vi "AttackHim.vi"(8 "error in (no error)":errorcluster, 9 "Cube":i32, 10 "Rival":refnum<class "Peasant.lvclass">, 11 "Peasant in":refnum<class "Peasant.lvclass">) -> (0 "error out":errorcluster, 1 "CurrentAttack":i32, 2 "Rival out":refnum<class "Peasant.lvclass">, 3 "Peasant out":refnum<class "Peasant.lvclass">)   [LabVIEW 2021, in "Peasant.lvclass"]
uses:
  Peasant.lvclass
  Peasant.lvclass/Peasant.ctl
  Accessory/Accessory.lvclass
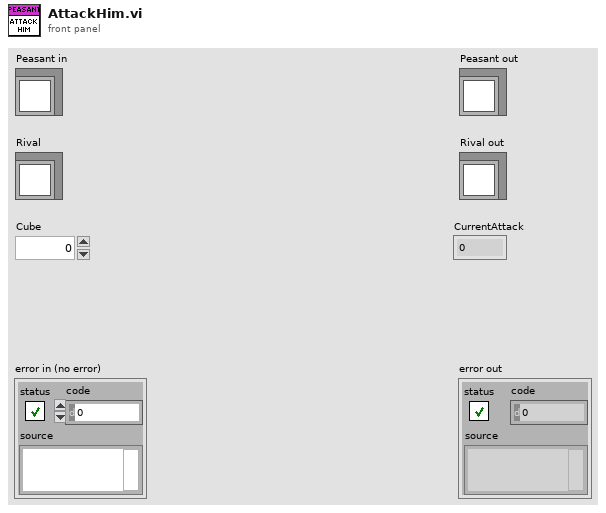
[diagram p1: front panel]
types:
  T1 = typedef "Peasant.lvclass/PeasantAttributes.ctl" = cluster{"Health":i32, "Stamina":i32, "Attack":i32, "Defense":i32, "Sing":i32}
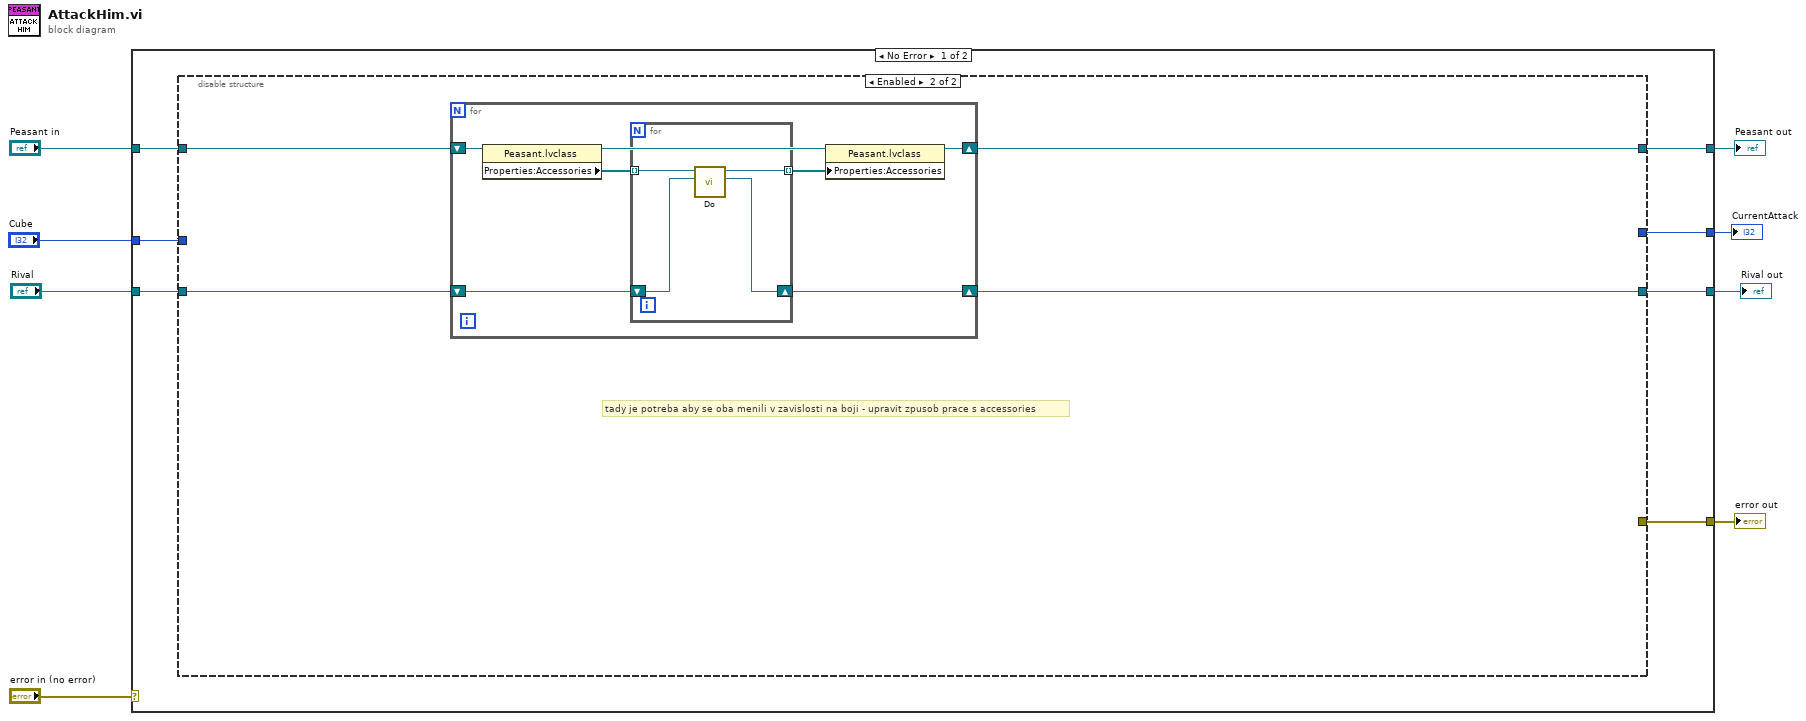
[diagram p0: block diagram]
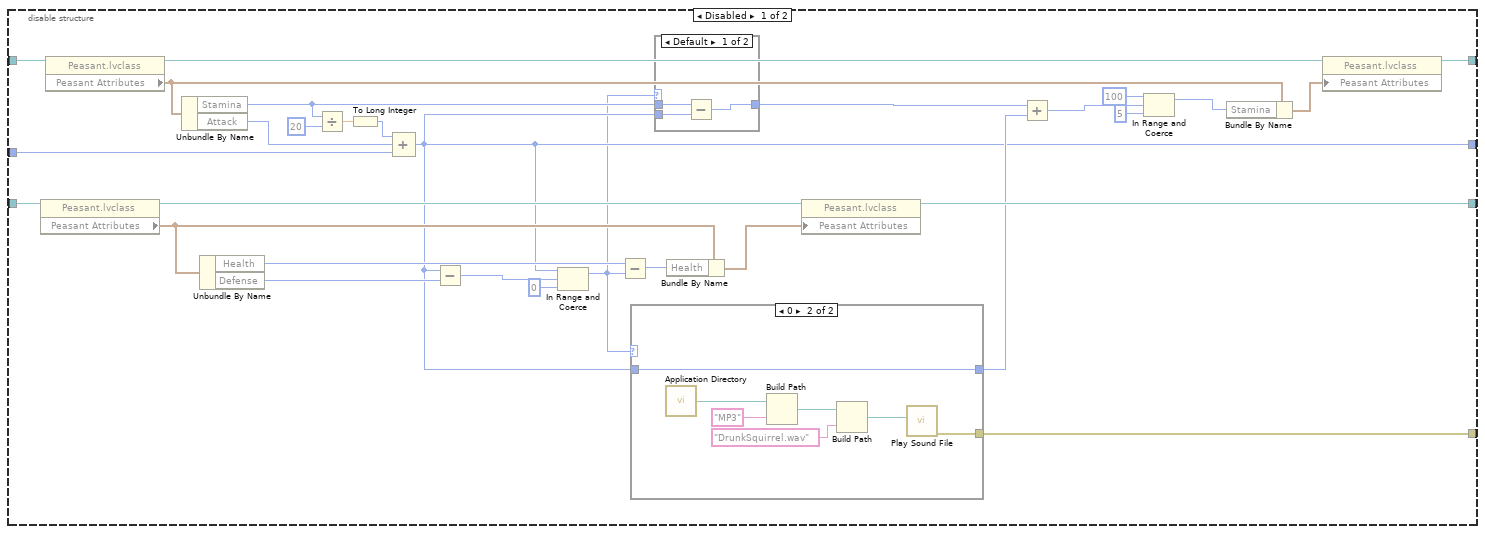
[diagram p2: hidden frame]
diagram:
  n1 = case shown="No Error" "error in (no error)" {
    selector: "error in (no error)" -> [_ w74]
    tunnel: [w11 w74] -> w7
    tunnel: [w12 w73] -> w5
    tunnel: "Peasant in" -> [w15 w73]
    tunnel: "Rival" -> [w14 w72]
    tunnel: "Cube" -> [w10 _]
    tunnel: [w13 w72] -> w2
    tunnel: [w9 _] -> w1
    frame No Error {
      n2 = disable-structure shown="Enabled" {
        disable-tunnel: w15 -> [w45 w60]
        disable-tunnel: w14 -> [w44 w59]
        disable-tunnel: [w38 w58] -> w13
        disable-tunnel: [w31 w57] -> w12
        disable-tunnel: [w30 _] -> w11
        disable-tunnel: w10 -> [w23 _]
        disable-tunnel: [w18 _] -> w9
        frame Disabled {
          n3 = property class="Peasant.lvclass"(reference=w44) -> (reference out=w40:refnum<class "Peasant.lvclass">, "Peasant Attributes"=w42:T1)  [unwired: 1 in, 1 out]
          n4 = property class="Peasant.lvclass"(reference=w45) -> (reference out=w34:refnum<class "Peasant.lvclass">, "Peasant Attributes"=w33:T1)  [unwired: 1 in, 1 out]
          n5 = Unbundle By Name(w33) -> ("Stamina"=w22:i32, "Attack"=w24:i32)
          n6 = Unbundle By Name(w42) -> ("Health"=w43:i32, "Defense"=w37:i32)
          n7 = Divide(x=w22, y=20) -> (x/y=w20:dbl)
          n8 = To Long Integer(number=w20) -> (32bit integer=w19:i32)
          n9 = Compound Arithmetic op=ADD(w19, w24, w23) -> (w18:i32)
          n10 = Subtract(x=w18, y=w37) -> (x-y=w35:i32)
          n11 = In Range and Coerce(upper limit=w18, x=w35, lower limit=0) -> (coerced(x)=w16:i32)  [unwired: 1 out]
          n12 = Subtract(x=w43, y=w16) -> (x-y=w41:i32)
          n13 = case shown="0" w16 {
            tunnel: [_ w51] -> w30
            tunnel: w18 -> [_ w50]
            tunnel: [_ w50] -> w28
            frame Default {
            }
            frame 0 {
              n14 = call <vilib>:"Application Directory.vi"() -> ("Application Directory"=w56:path)
              n15 = Build Path(base path=w56, name or relative path="MP3") -> (appended path=w54:path)
              n16 = Build Path(base path=w54, name or relative path="DrunkSquirrel.wav") -> (appended path=w52:path)
              n17 = call <vilib>:"Play Sound File.vi"("path"=w52) -> ("error out"=w51:errorcluster)  [unwired: 9 in, 1 out]
            }
          }
          n18 = case shown="Default" w16 {
            tunnel: [w48 w49] -> w29
            tunnel: w22 -> [w47 w49]
            tunnel: w18 -> [w46 _]
            frame Default {
              n19 = Subtract(x=w47, y=w46) -> (x-y=w48:i32)
            }
            frame 0 {
            }
          }
          n20 = Bundle By Name(cluster=w42, "Health"=w41) -> (w39:T1)
          n21 = property class="Peasant.lvclass"(reference=w40, "Peasant Attributes"=w39) -> (reference out=w38:refnum<class "Peasant.lvclass">)  [unwired: 1 in, 1 out]
          n22 = Add(x=w29, y=w28) -> (x+y=w27:i32)
          n23 = In Range and Coerce(upper limit=100, x=w27, lower limit=5) -> (coerced(x)=w25:i32)  [unwired: 1 out]
          n24 = Bundle By Name(cluster=w33, "Stamina"=w25) -> (w32:T1)
          n25 = property class="Peasant.lvclass"(reference=w34, "Peasant Attributes"=w32) -> (reference out=w31:refnum<class "Peasant.lvclass">)  [unwired: 1 in, 1 out]
        }
        frame Enabled {
          # "tady je potreba aby se oba menili v zavislosti na boji - upravit zpusob prace s accessories"
          n26 = for {
            shift-right: [w66] -> w58
            shift-left: w59 -> [w67]
            shift-right: [w62] -> w57
            shift-left: w60 -> [w65]
            n27 = property class="Peasant.lvclass"(reference=w65) -> (reference out=w63:refnum<class "Peasant.lvclass">, "Properties:Accessories"=w64:refnum<class "Accessory.lvclass">[])  [unwired: 1 in, 1 out]
            n28 = for {
              shift-right: [w70] -> w66
              shift-left: w67 -> [w71]
              tunnel: w64 -> [w69] mode=indexing
              tunnel: [w68] -> w61 mode=indexing
              n29 = call-dynamic "Do.vi"("Rival"=w71, "Accessory in"=w69) -> ("Rival"=w70:refnum<class "Peasant.lvclass">, "Accessory out"=w68:refnum<class "Accessory.lvclass">)  [unwired: 7 in, 1 out]
            }
            n30 = property class="Peasant.lvclass"(reference=w63, "Properties:Accessories"=w61) -> (reference out=w62:refnum<class "Peasant.lvclass">)  [unwired: 1 in, 1 out]
          }
        }
      }
    }
    frame Error {
    }
  }
  "error out" <- w7
  "Peasant out" <- w5
  "Rival out" <- w2
  "CurrentAttack" <- w1
